vi "Test Server.vi"() -> ()   [LabVIEW 2020]
uses:
  source/Value/Value/Value.lvclass
  source/Server/Server/Server.lvclass
  source/Server/Source/Source.lvclass
  source/Value/Value.lvlib
  67596c9d-494e-4045-aa1e-399bd9a06ed6.vi
  41ac7609-5d0e-48bc-9034-e5839c72e2f8.vi
  b4702106-43b1-43e1-a377-b71557efabfc.vi
  source/Value/Type Code.ctl
  Every Type Code.ctl
  source/Value/Value Fields.ctl
  f4a45bcd-a069-4b90-ba05-607c19a46b76.vi
  <vilib>/numeric/Random Number (Range) I64.vi
panel:
  out "value":variant
  out "timestamp":timestamp
  in  "PV":u16(ring) items=["BOOL", "INT8", "INT16", "INT32", "INT64", "UINT8", "UINT16", "UINT32", "UINT64", "FLOAT32", "FLOAT64", "STRING", "BOOL_ARRAY", "INT8_ARRAY", "INT16_ARRAY", "INT32_ARRAY", "INT64_ARRAY", "UINT8_ARRAY", "UINT16_ARRAY", "UINT32_ARRAY", "UINT64_ARRAY", "FLOAT32_ARRAY", "FLOAT64_ARRAY", "STRING_ARRAY"]
  in  "Update":bool caption="Update values"
  in  "stop":bool
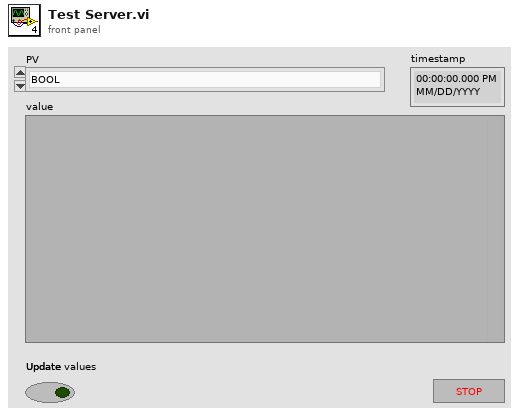
[diagram p1: front panel]
types:
  T1 = typedef "Value.lvlib/Value Fields.ctl" = cluster{"Display":bool, "Control":bool, "Value alarm":bool}
  T2 = typedef "Every Type Code.ctl" = T3[]
  T3 = typedef "Value.lvlib/Type Code.ctl" = enum8{"Null", "Bool", "BoolA", "Int8", "Int8A", "Int16", "Int16A", "Int32", "Int32A", "Int64", "Int64A", "UInt8", "UInt8A", "UInt16", "UInt16A", "UInt32", "UInt32A", "UInt64", "UInt64A", "Float32", "Float32A", "Float64", "Float64A", "String", "StringA", "Struct", "StructA", "Union", "UnionA", "Any", "AnyA"}
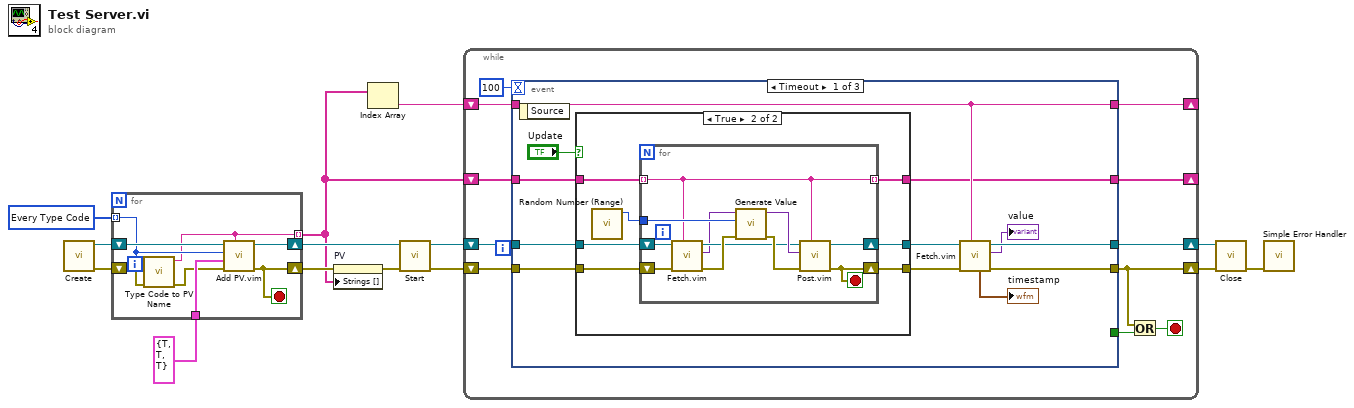
[diagram p0: block diagram]
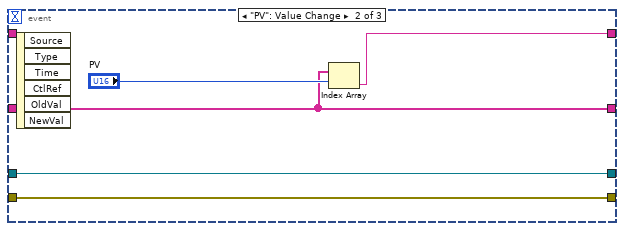
[diagram p3: hidden frame]
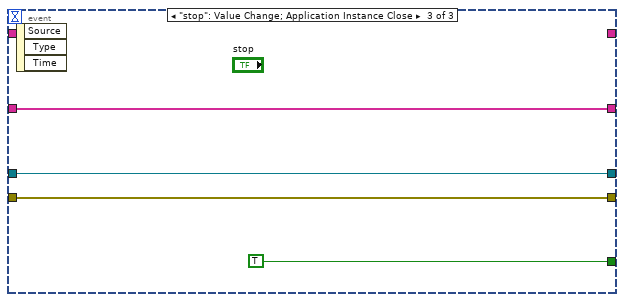
[diagram p4: hidden frame]
diagram:
  w5 = T2 [enum."Bool", enum."Int8", enum."Int16", enum."Int32", enum."Int64", enum."UInt8", enum."UInt16", enum."UInt32", enum."UInt64", enum."Float32", enum."Float64", enum."String", enum."BoolA", enum."Int8A", enum."Int16A", enum."Int32A", enum."Int64A", enum."UInt8A", enum."UInt16A", enum."UInt32A", enum."UInt64A", enum."Float32A", enum."Float64A", enum."StringA"] items=["Null", "Bool", "BoolA", "Int8", "Int8A", "Int16", "Int16A", "Int32", "Int32A", "Int64", "Int64A", "UInt8", "UInt8A", "UInt16", "UInt16A", "UInt32", "UInt32A", "UInt64", "UInt64A", "Float32", "Float32A", "Float64", "Float64A", "String", "StringA", "Struct", "StructA", "Union", "UnionA", "Any", "AnyA"] ("Array")
  n1 = call "Create.vi"() -> ("error out"=w11:errorcluster, "Server out"=w10:refnum<class "Server.lvclass">)  [unwired: 10 in]
  n2 = for {
    shift-right: [w22] -> w12
    shift-left: w10 -> [w19]
    tunnel: [w15] -> w1 mode=indexing
    shift-right: [w21] -> w3
    shift-left: w11 -> [w20]
    tunnel: T1 {"Display"=TRUE, "Control"=TRUE, "Value alarm"=TRUE} ("fields") -> [w17]
    tunnel: w5 -> [w18] mode=indexing
    stop <- w21 stop-if-true
    n3 = call "Type Code to PV Name.vi"("error in (no error)"=w20, "type code"=w18) -> ("error out"=w16:errorcluster, "PV name"=w15:string)  [unwired: 8 in]
    n4 = call "Add PV.vim"("PV name"=w15, "error in"=w16, "fields"=w17, "initial value"=w18, "Server in"=w19) -> ("error out"=w21:errorcluster, "Server out"=w22:refnum<class "Server.lvclass">)  [unwired: 3 in, 2 out]
  }
  n5 = property on="PV" class="Ring (strict)"(error in=w3, "Strings []"=w1) -> (error out=w2:errorcluster)  [unwired: 1 in, 1 out]
  n6 = Index Array(array=w1) -> (element=w4:string)  [unwired: 1 in]
  n7 = call-dynamic "Start.vi"("error in (no error)"=w2, "Server in"=w12) -> ("error out"=w14:errorcluster, "Server out"=w13:refnum<class "Server.lvclass">)  [unwired: 8 in]
  n8 = while {
    shift-right: [w28] -> w9
    shift-left: w14 -> [w33]
    shift-right: [w31] -> w8
    shift-left: w13 -> [w32]
    shift-right: [w25] -> _
    shift-left: w1 -> [w26]
    shift-right: [w24] -> _
    shift-left: w4 -> [w23]
    stop <- w30 stop-if-true
    n9 = event shown="[0] Timeout" {
      selector: _ -> [_ _ _]
      dyn-events: _ -> [_ _ _]
      timeout: 100 -> [_ _ _]
      tunnel: [w38 w70 w75] -> w28
      tunnel: w33 -> [w44 w70 w75]
      tunnel: w32 -> [w45 w71 w74]
      tunnel: [w39 w71 w74] -> w31
      tunnel: [_ _ TRUE] -> w29
      tunnel: w26 -> [w42 w67 w72]
      tunnel: [w34 w67 w72] -> w25
      tunnel: [w37 w68 _] -> w24
      tunnel: w23 -> [w37 _ _]
      event Timeout {
        n10 = event-data() -> ()  [unwired: 1 in, 1 out]
        n11 = case shown="True" "Update" {
          tunnel: w45 -> [w48 w55]
          tunnel: [w48 w54] -> w40
          tunnel: w44 -> [w47 w53]
          tunnel: [w47 w52] -> w41
          tunnel: w42 -> [w46 w50]
          tunnel: [w46 w49] -> w34
          frame False {
          }
          frame True {
            n12 = call-poly <vilib>:"Random Number (Range).vi"() -> ("number"=w51:i64)  [unwired: 11 in]
            n13 = for {
              shift-right: [w64] -> w52
              shift-left: w53 -> [w61]
              tunnel: w50 -> [w56] mode=indexing
              shift-right: [w66] -> w54
              shift-left: w55 -> [w59]
              tunnel: w51 -> [w65]
              tunnel: [w56] -> w49 mode=indexing
              stop <- w64 stop-if-true
              n14 = call "Fetch.vim"("PV name"=w56, "error in"=w61, "Server in"=w59) -> ("error out"=w60:errorcluster, "value"=w57:variant, "Server out"=w58:refnum<class "Server.lvclass">)  [unwired: 5 in, 1 out]
              n15 = call "Generate Value.vi"("error in (no error)"=w60, "base value"=w65, "variant"=w57) -> ("error out"=w62:errorcluster, "value"=w63:variant)  [unwired: 7 in]
              n16 = call "Post.vim"("PV name"=w56, "error in"=w62, "value in"=w63, "Server in"=w58) -> ("error out"=w64:errorcluster, "Server out"=w66:refnum<class "Server.lvclass">)  [unwired: 5 in, 1 out]
            }
          }
        }
        n17 = call "Fetch.vim"("PV name"=w37, "error in"=w41, "Server in"=w40) -> ("error out"=w38:errorcluster, "value"=→"value":variant, "Server out"=w39:refnum<class "Server.lvclass">, "timestamp"=→"timestamp":timestamp)  [unwired: 5 in]
      }
      event "PV": Value Change {
        n18 = event-data() -> ()  [unwired: 1 in, 6 out]
        n19 = Index Array(array=w67, index="PV") -> (element=w68:string)
      }
      event "stop": Value Change; Application Instance Close {
        n20 = event-data() -> ()  [unwired: 1 in, 3 out]
      }
    }
    n21 = Or(x=w28, y=w29) -> (x .or. y?=w30:bool)
  }
  n22 = call-dynamic "Close.vi"("error in"=w9, "Server in"=w8) -> ("error out"=w7:errorcluster)  [unwired: 9 in]
  n23 = call <vilib>:"Simple Error Handler.vi"("error in (no error)"=w7) -> ()  [unwired: 4 in, 5 out]
